vi "Heater controll.vi"() -> (0 "MANUAL HEATER DISPLAY":dbl(slide) caption="AMP" min=0.0 max=99.0 scale=0.0..5.0, 1 "Heater DIsplay":bool[](array[boolean]), 2 "HEATER ON":bool)   [LabVIEW 2019]
uses:
  GL_MHeaterDisplay.vi
  GL_heaterdisplay.vi
  GL_HeaterOn.vi
panel:
  out "Manual Heater on":bool
  in  "Manual Heater on":bool
  out "MANUAL HEATER SETTING":dbl format="%.2f"
  in  "CLOSE":bool
  in  "MANUAL HEATER":dbl(slide) caption="AMP" min=0.0 max=990.0 scale=0.0..5.0
  out "HEATER RANGE":dbl format="%.2f"
  out "Change state bit":bool
  in  "Heater Input":bool[](array[boolean])
  # "0/1 -4  -3   -2   -1   M"
  # "MANUAL HEATER"
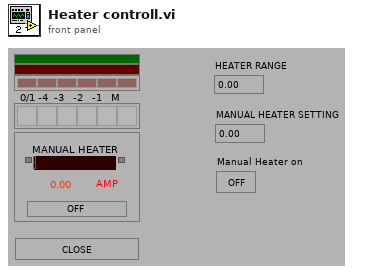
[diagram p1: front panel]
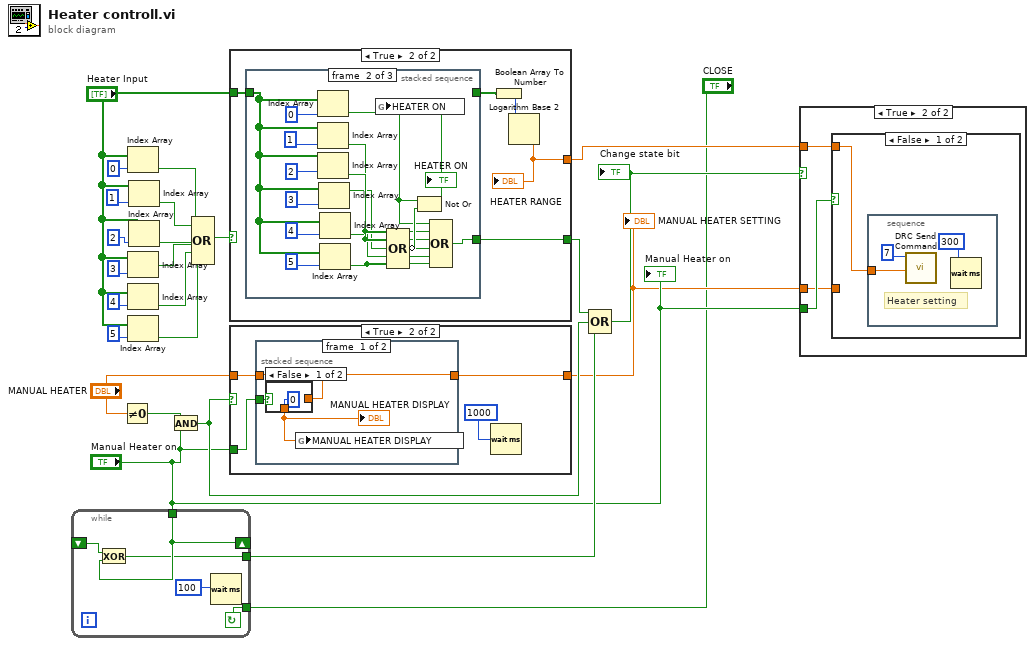
[diagram p0: block diagram]
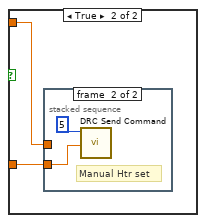
[diagram p3: hidden frame]
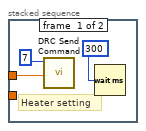
[diagram p4: hidden frame]
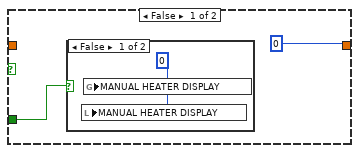
[diagram p5: hidden frame]
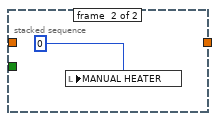
[diagram p8: hidden frame]
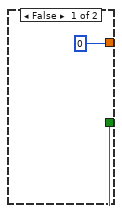
[diagram p9: hidden frame]
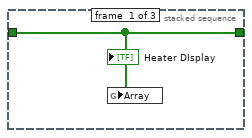
[diagram p10: hidden frame]
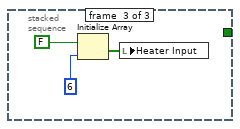
[diagram p11: hidden frame]
diagram:
  n1 = while {
    tunnel: "CLOSE" -> [w25]
    tunnel: [w26] -> w9
    tunnel: "Manual Heater on" -> [w27]
    shift-left: _ -> [w29]
    shift-right: [w27] -> _
    stop <- w25 continue-if-true
    n2 = Exclusive Or(1:w27, 2:w29) -> (0:w26:bool)
    n3 = Wait (ms)(milliseconds to wait=100) -> ()  [unwired: 1 out]
  }
  n4 = Not Equal To 0?(x="MANUAL HEATER") -> (x != 0?=w11:bool)
  n5 = Index Array(array="Heater Input", index=0) -> (element=w18:bool)
  n6 = Index Array(array="Heater Input", index=3) -> (element=w15:bool)
  n7 = Index Array(array="Heater Input", index=4) -> (element=w1:bool)
  n8 = Index Array(array="Heater Input", index=5) -> (element=w2:bool)
  n9 = Index Array(array="Heater Input", index=1) -> (element=w17:bool)
  n10 = Index Array(array="Heater Input", index=2) -> (element=w16:bool)
  n11 = And(x=w11, y="Manual Heater on") -> (x .and. y?=w10:bool)
  n12 = Compound Arithmetic op=OR(w18, w17, w16, w15, w1, w2) -> (w19:bool)
  n13 = case shown="True" w19 {
    tunnel: "Heater Input" -> [_ w36]
    tunnel: [FALSE w33] -> w12
    tunnel: [0 w32] -> w7
    frame False {
    }
    frame True {
      n14 = stacked-sequence {
        tunnel: w36 -> [w37 w41 _]
        tunnel: [_ w46 _] -> w33
        tunnel: [w37 _ _] -> w35
        frame #0 {
          n15 = global write "GL_heaterdisplay.vi" "Array"(w37) -> ()
          "Heater DIsplay" <- w37
        }
        frame #1 {
          n16 = Index Array(array=w41, index=0) -> (element=w43:bool)
          n17 = Index Array(array=w41, index=1) -> (element=w44:bool)
          n18 = Index Array(array=w41, index=2) -> (element=w45:bool)
          n19 = Index Array(array=w41, index=3) -> (element=w40:bool)
          n20 = Index Array(array=w41, index=4) -> (element=w38:bool)
          n21 = Index Array(array=w41, index=5) -> (element=w39:bool)
          n22 = Compound Arithmetic op=OR(w44, w45, w40, w38, w39) -> (invert w49:bool)
          n23 = Not Or(1:w49, 2:w43) -> (0:w48:bool)
          "HEATER ON" <- w48
          n24 = global write "GL_HeaterOn.vi" "HEATER ON"(w48) -> ()
          n25 = Compound Arithmetic op=OR(w43, w44, w45, w40, w38, w39) -> (w46:bool)
        }
        frame #2 {
          n26 = Initialize Array(FALSE, 6) -> (w55:bool[])
          n27 = local write "Heater Input"(w55) -> ()
        }
      }
      n28 = Boolean Array To Number(Boolean array=w35) -> (number=w34:u32)
      n29 = Logarithm Base 2(1:w34) -> (0:w32:dbl)
      "HEATER RANGE" <- w32
    }
  }
  n30 = case shown="True" w10 {
    tunnel: "MANUAL HEATER" -> [_ w63]
    tunnel: [0 w62] -> w6
    tunnel: "Manual Heater on" -> [w57 w60]
    frame False {
      n31 = case shown="False" w57 {
        frame False {
          w59 = 0
          n32 = local write "MANUAL HEATER DISPLAY"(w59) -> ()
          n33 = global write "GL_MHeaterDisplay.vi" "MANUAL HEATER DISPLAY"(w59) -> ()
        }
        frame True {
        }
      }
    }
    frame True {
      n34 = stacked-sequence {
        tunnel: w63 -> [w66 _]
        tunnel: [w66 _] -> w62
        tunnel: w60 -> [w64 _]
        frame #0 {
          n35 = case shown="False" w64 {
            tunnel: [0 w68] -> w65
            tunnel: w66 -> [_ w68]
            frame False {
            }
            frame True {
            }
          }
          "MANUAL HEATER DISPLAY" <- w65
          n36 = global write "GL_MHeaterDisplay.vi" "MANUAL HEATER DISPLAY"(w65) -> ()
        }
        frame #1 {
          n37 = local write "MANUAL HEATER"(0) -> ()
        }
      }
      n38 = Wait (ms)(milliseconds to wait=1000) -> ()  [unwired: 1 out]
    }
  }
  "MANUAL HEATER SETTING" <- w6
  n39 = Compound Arithmetic op=OR(w12, w10, w9) -> (w13:bool)
  "Change state bit" <- w13
  n40 = case shown="True" w13 {
    tunnel: "Manual Heater on" -> [_ w71]
    tunnel: w7 -> [_ w72]
    tunnel: w6 -> [_ w70]
    frame False {
    }
    frame True {
      n41 = case shown="False" w71 {
        tunnel: w72 -> [w73 w78]
        tunnel: w70 -> [_ w77]
        frame False {
          n42 = stacked-sequence {
            tunnel: w73 -> [w75]
            frame #0 {
              # "Heater setting"
              n43 = call "DRC Send Command.vi"("Input"=w75, "Command"=7) -> ()  [unwired: 2 in, 3 out]
              n44 = Wait (ms)(milliseconds to wait=300) -> ()  [unwired: 1 out]
            }
          }
        }
        frame True {
          n45 = stacked-sequence {
            tunnel: w78 -> [w80 _]
            tunnel: w77 -> [_ w82]
            frame #0 {
              # "Heater setting"
              n46 = call "DRC Send Command.vi"("Input"=w80, "Command"=7) -> ()  [unwired: 2 in, 3 out]
              n47 = Wait (ms)(milliseconds to wait=300) -> ()  [unwired: 1 out]
            }
            frame #1 {
              # "Manual Htr set"
              n48 = call "DRC Send Command.vi"("Input"=w82, "Command"=5) -> ()  [unwired: 2 in, 3 out]
            }
          }
        }
      }
    }
  }
  "Manual Heater on" <- "Manual Heater on"
